vi "2D_Seven_Segment.vi"() -> ()   [LabVIEW 2024]
panel:
  in  "Numeric 2":i32
  out "Boolean 14":bool
  out "Boolean 13":bool
  out "Boolean 12":bool
  out "Boolean 11":bool
  out "Boolean 10":bool
  out "Boolean 9":bool
  out "Boolean 8":bool
  in  "Numeric":i32
  out "Boolean 4":bool
  out "Boolean 7":bool
  out "Boolean 3":bool
  out "Boolean 5":bool
  out "Boolean 6":bool
  out "Boolean 2":bool
  out "Boolean 1":bool
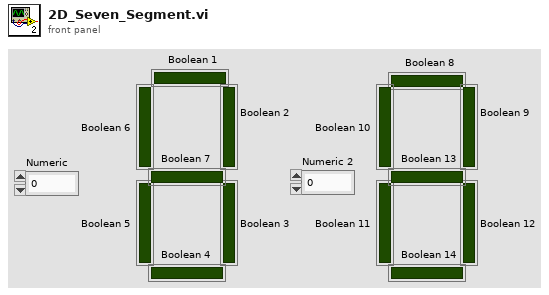
[diagram p1: front panel]
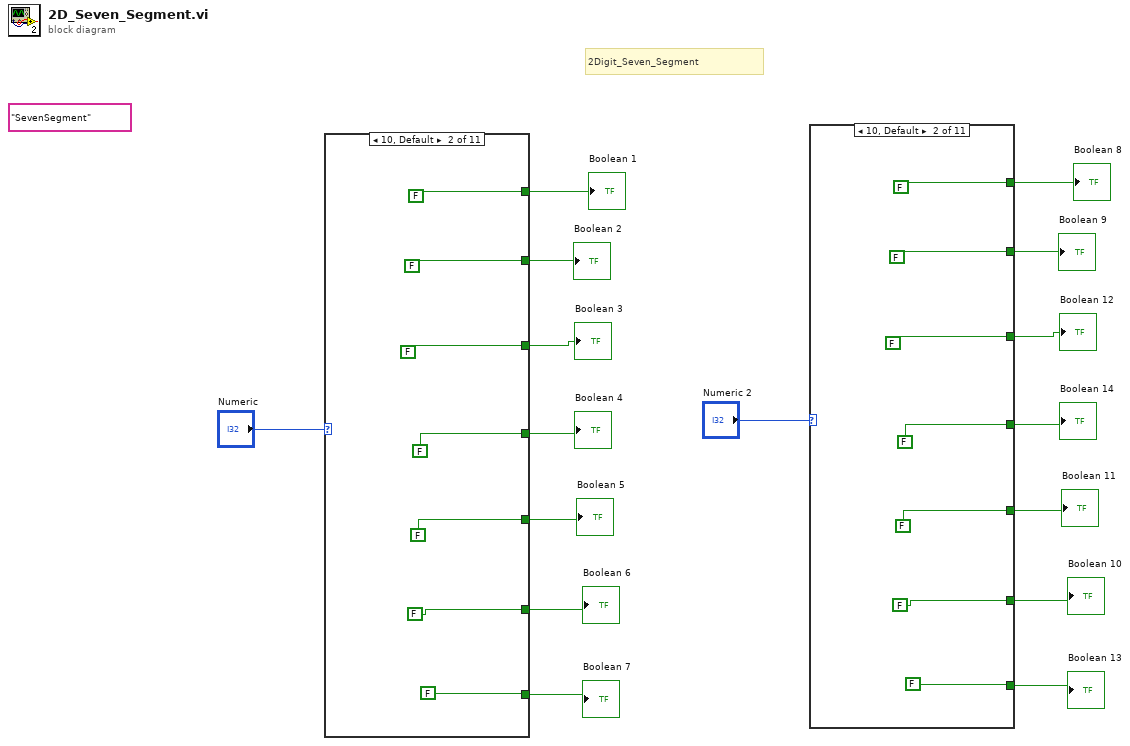
[diagram p0: block diagram]
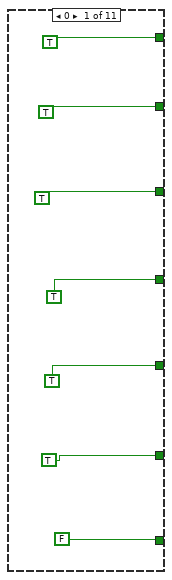
[diagram p2: hidden frame]
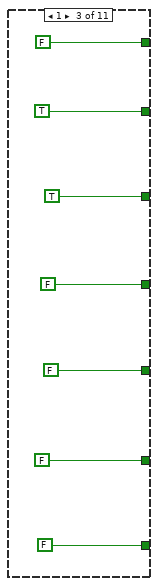
[diagram p3: hidden frame]
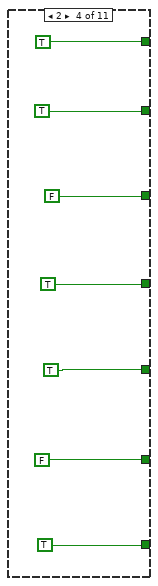
[diagram p4: hidden frame]
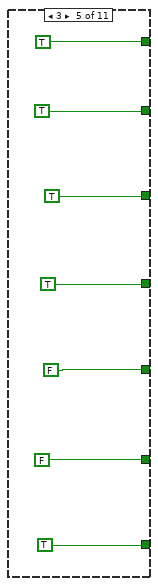
[diagram p5: hidden frame]
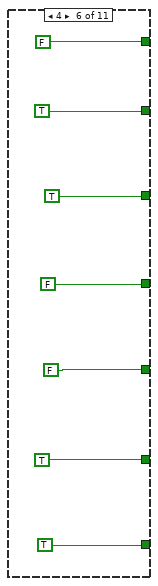
[diagram p6: hidden frame]
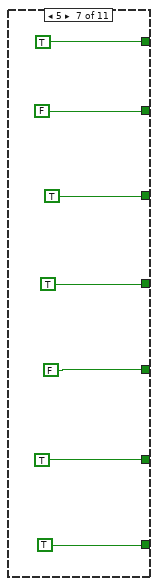
[diagram p7: hidden frame]
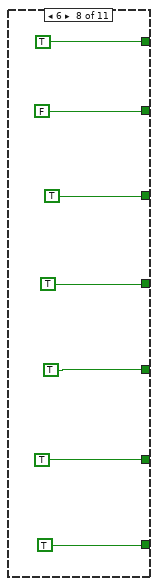
[diagram p8: hidden frame]
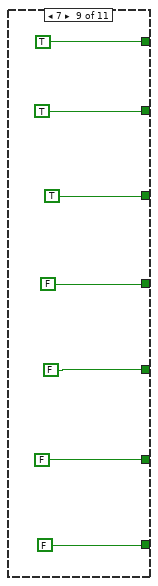
[diagram p9: hidden frame]
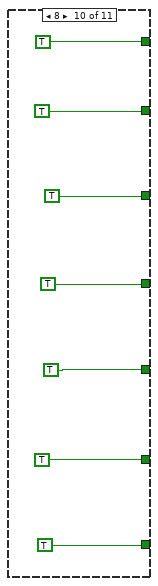
[diagram p10: hidden frame]
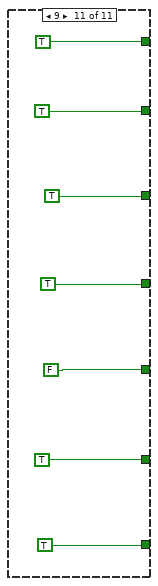
[diagram p11: hidden frame]
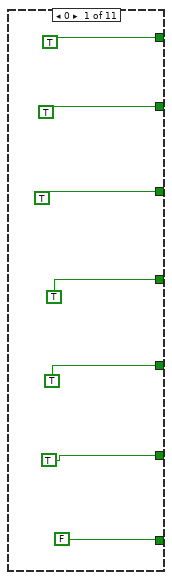
[diagram p12: hidden frame]
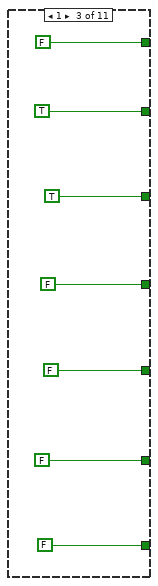
[diagram p13: hidden frame]
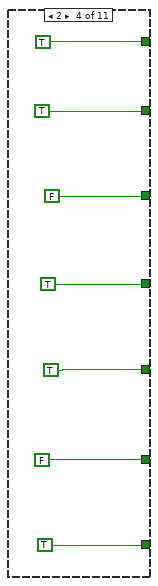
[diagram p14: hidden frame]
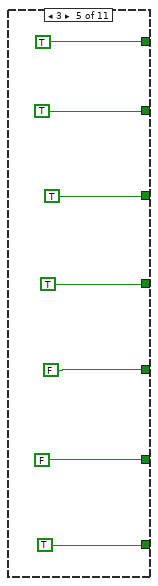
[diagram p15: hidden frame]
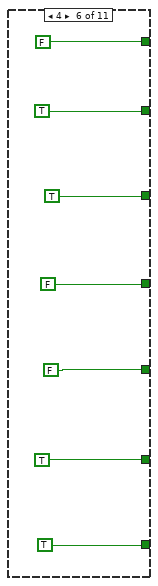
[diagram p16: hidden frame]
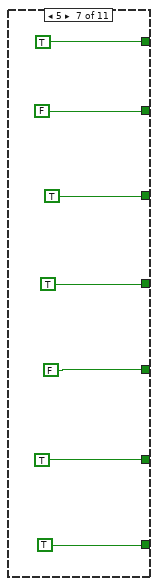
[diagram p17: hidden frame]
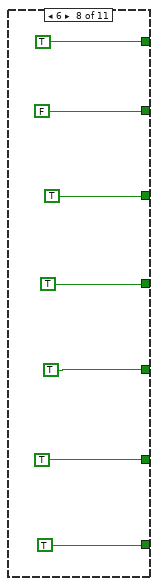
[diagram p18: hidden frame]
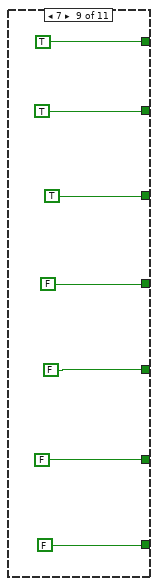
[diagram p19: hidden frame]
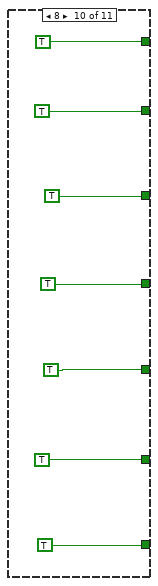
[diagram p20: hidden frame]
diagram:
  (unwired) "SevenSegment"
  # "2Digit_Seven_Segment"
  n1 = case shown="10, Default" "Numeric" {
    tunnel: [TRUE FALSE FALSE TRUE TRUE FALSE TRUE TRUE TRUE TRUE TRUE] -> w16
    tunnel: [TRUE FALSE TRUE TRUE TRUE TRUE FALSE FALSE TRUE TRUE TRUE] -> w15
    tunnel: [TRUE FALSE TRUE FALSE TRUE TRUE TRUE TRUE TRUE TRUE TRUE] -> w14
    tunnel: [TRUE FALSE FALSE TRUE TRUE FALSE TRUE TRUE FALSE TRUE TRUE] -> w13
    tunnel: [TRUE FALSE FALSE TRUE FALSE FALSE FALSE TRUE FALSE TRUE FALSE] -> w12
    tunnel: [TRUE FALSE FALSE FALSE FALSE TRUE TRUE TRUE FALSE TRUE TRUE] -> w11
    tunnel: [FALSE FALSE FALSE TRUE TRUE TRUE TRUE TRUE FALSE TRUE TRUE] -> w10
    frame 0 {
    }
    frame 10, Default {
    }
    frame 1 {
    }
    frame 2 {
    }
    frame 3 {
    }
    frame 4 {
    }
    frame 5 {
    }
    frame 6 {
    }
    frame 7 {
    }
    frame 8 {
    }
    frame 9 {
    }
  }
  "Boolean 1" <- w16
  "Boolean 2" <- w15
  "Boolean 6" <- w11
  "Boolean 5" <- w12
  "Boolean 3" <- w14
  "Boolean 7" <- w10
  "Boolean 4" <- w13
  n2 = case shown="10, Default" "Numeric 2" {
    tunnel: [TRUE FALSE FALSE TRUE TRUE FALSE TRUE TRUE TRUE TRUE TRUE] -> w8
    tunnel: [TRUE FALSE TRUE TRUE TRUE TRUE FALSE FALSE TRUE TRUE TRUE] -> w7
    tunnel: [TRUE FALSE TRUE FALSE TRUE TRUE TRUE TRUE TRUE TRUE TRUE] -> w6
    tunnel: [TRUE FALSE FALSE TRUE TRUE FALSE TRUE TRUE FALSE TRUE TRUE] -> w5
    tunnel: [TRUE FALSE FALSE TRUE FALSE FALSE FALSE TRUE FALSE TRUE FALSE] -> w4
    tunnel: [TRUE FALSE FALSE FALSE FALSE TRUE TRUE TRUE FALSE TRUE TRUE] -> w3
    tunnel: [FALSE FALSE FALSE TRUE TRUE TRUE TRUE TRUE FALSE TRUE TRUE] -> w2
    frame 0 {
    }
    frame 10, Default {
    }
    frame 1 {
    }
    frame 2 {
    }
    frame 3 {
    }
    frame 4 {
    }
    frame 5 {
    }
    frame 6 {
    }
    frame 7 {
    }
    frame 8 {
    }
    frame 9 {
    }
  }
  "Boolean 8" <- w8
  "Boolean 9" <- w7
  "Boolean 10" <- w3
  "Boolean 11" <- w4
  "Boolean 12" <- w6
  "Boolean 13" <- w2
  "Boolean 14" <- w5
